vi "Write irqHandler.vi"(10 "irqHandler":refnum<class "IIRQHandler.lvclass">, 11 "CompactRIO in":refnum<class "CompactRIO.lvclass">) -> (3 "CompactRIO out":refnum<class "CompactRIO.lvclass">)   [LabVIEW 2012, in "CompactRIO.lvclass"]
uses:
  CompactRIO.lvclass
  C/Program Files (x86)/National Instruments/LabVIEW 2012/user.lib/Common/ComponentModel/ComponentModelRT/IRQHandler/IIRQHandler/IIRQHandler.lvclass
  CompactRIO.lvclass/CompactRIO.ctl
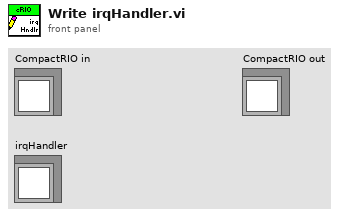
[diagram p1: front panel]
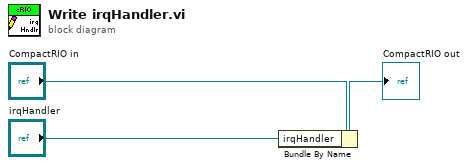
[diagram p0: block diagram]
diagram:
  n1 = Bundle By Name(cluster="CompactRIO in", "irqHandler"="irqHandler") -> (→"CompactRIO out":refnum<class "CompactRIO.lvclass">)
